vi "Add Comparator Item to Tree.vi"(6 "Connected?":bool, 8 "error in (no error)":errorcluster, 9 "Name in":string, 10 "Tag":string, 11 "TreeControl in":refnum<vi>) -> (0 "error out":errorcluster, 2 "Comparator Tag out":string, 3 "TreeControl out":refnum<vi>)   [LabVIEW 2018, in "Test Manager.lvlib"]
uses:
  Test Manager.lvlib
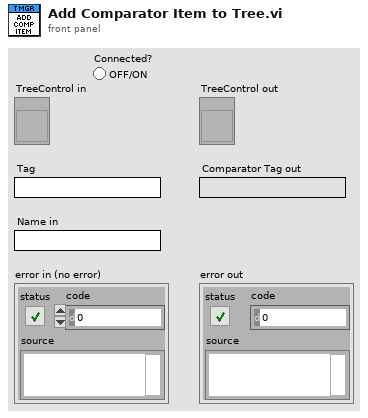
[diagram p1: front panel]
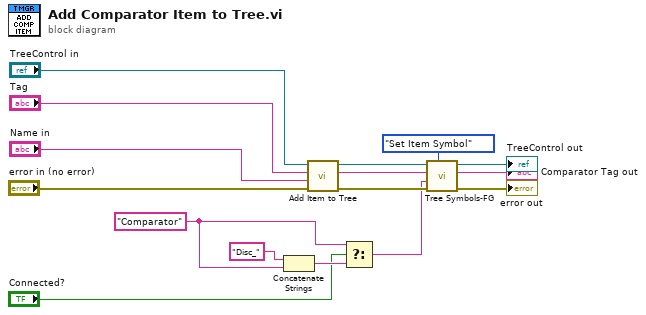
[diagram p0: block diagram]
diagram:
  w3 = "Comparator" ("Symbol Name")
  n1 = Concatenate Strings("Disc_" ("string"), w3) -> (w4:string)
  n2 = call "Add Item to Tree.vi"("error in (no error)"="error in (no error)", "Item Name"="Name in", "Item Tag"="Tag", "Tree Ref"="TreeControl in") -> ("error out"=w11:errorcluster, "Item Tag out"=w13:string, "reference out"=w12:refnum<vi>)  [unwired: 4 in, 1 out]
  n3 = Select(t=w3, s="Connected?", f=w4) -> (s? t:f=w1:string)
  n4 = call "Tree Symbols-FG.vi"("Actions"=enum16{"Init Symbols", "Set Item Symbol"}."Set Item Symbol", "error in (no error)"=w11, "Symbol Name"=w1, "Item Tag"=w13, "Tree Ref"=w12) -> ("error out"=→"error out":errorcluster, "Item Tag out"=→"Comparator Tag out":string, "Tree Ref out"=→"TreeControl out":refnum<vi>)  [unwired: 4 in]
